vi "PRL TS Waiter.vi"(11 "Ms to Wait":u32) -> (3 "Trigger?":bool)   [LabVIEW 2013, in "PMU Recorder Light.lvlib"]
uses:
  PMU Recorder Light.lvlib
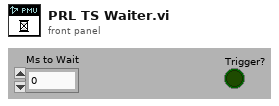
[diagram p1: front panel]
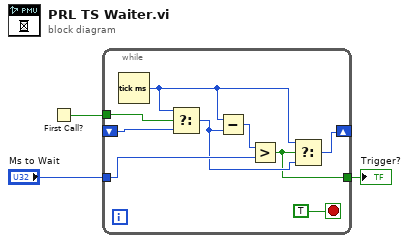
[diagram p0: block diagram]
diagram:
  n1 = First Call?() -> (First Call?: T/F=w1:bool)
  n2 = while {
    shift-right: [w6] -> _
    shift-left: _ -> [w10]
    tunnel: w1 -> [w11]
    tunnel: "Ms to Wait" -> [w8]
    tunnel: [w4] -> w2
    stop <- TRUE stop-if-true
    n3 = Tick Count (ms)() -> (millisecond timer value=w7:u32)
    n4 = Select(t=w7, s=w11, f=w10) -> (s? t:f=w5:u32)
    n5 = Subtract(x=w7, y=w5) -> (x-y=w9:u32)
    n6 = Greater?(x=w9, y=w8) -> (0:w4:bool)
    n7 = Select(t=w7, s=w4, f=w5) -> (s? t:f=w6:u32)
  }
  "Trigger?" <- w2
